vi "MenuDropdown.vi"(8 "error in (no error)":errorcluster) -> (0 "error out":errorcluster)   [LabVIEW 2019, in "MenuDropdown.lvlib"]
uses:
  MenuDropdown.lvlib
panel:
  in  "MenuItems":bool[](array[boolean])
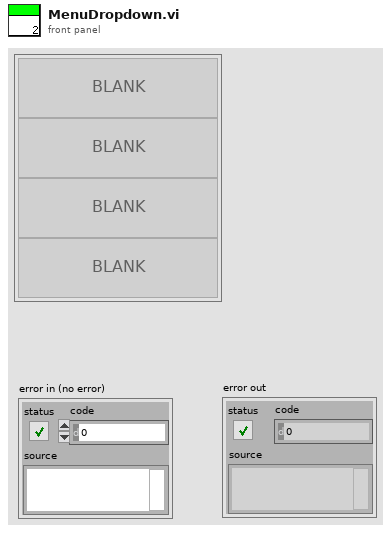
[diagram p1: front panel]
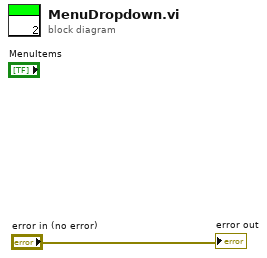
[diagram p0: block diagram]
diagram:
  "error out" <- "error in (no error)"
